vi "MicronClient.vi"() -> ()   [LabVIEW 2019]
uses:
  <vilib>/SLL Toolkit/SLL Easy TCP/_SubVIs/TCP Initialize Client - Local.vi
  <vilib>/SLL Toolkit/SLL Easy TCP/SLL Easy API via TCP.lvclass
panel:
  in  "Command":string(combo)="Ping"
  out "error out":errorcluster
  out "Read Data":string
  in  "Service Name":string="Micron-1"
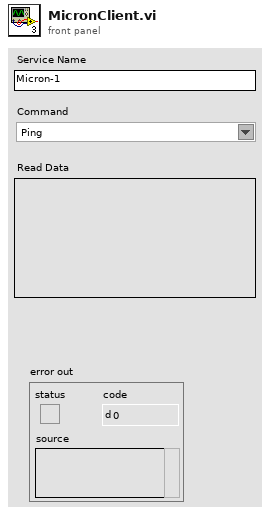
[diagram p1: front panel]
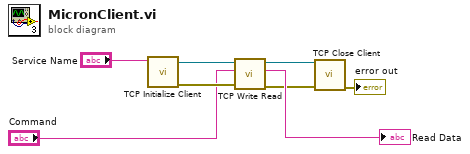
[diagram p0: block diagram]
diagram:
  n1 = call-poly <vilib>:"TCP Initialize Client.vi"("Service Name"="Service Name") -> ("error out"=w5:errorcluster, "connection ID Out"=w8:refnum<k5>)  [unwired: 9 in]
  n2 = call <vilib>:"TCP Write Read.vi"("error in (no error)"=w5, "Write Data"="Command", "connection ID In"=w8) -> ("error out"=w4:errorcluster, "Read Data"=→"Read Data":string, "connection ID Out"=w7:refnum<k5>)  [unwired: 5 in, 1 out]
  n3 = call <vilib>:"TCP Close Client.vi"("error in (no error)"=w4, "connection ID"=w7) -> ("error out"=→"error out":errorcluster)  [unwired: 9 in]
